vi "JSON_Mass_Find (SubVI).vi"(10 "Array in":string[](array[string]), 11 "Param":string) -> (3 "Array out":string[](array[string]))   [LabVIEW 2018]
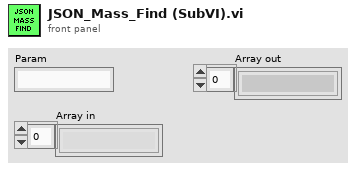
[diagram p1: front panel]
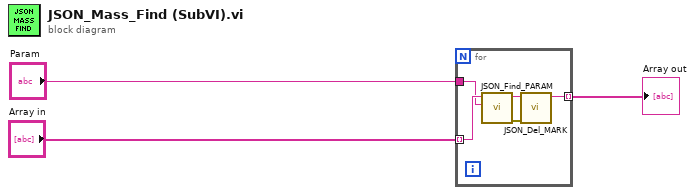
[diagram p0: block diagram]
diagram:
  n1 = for {
    tunnel: "Array in" -> [w8] mode=indexing
    tunnel: [w5] -> w2 mode=indexing
    tunnel: "Param" -> [w4]
    n2 = call "JSON_Find_PARAM.vi"("data"=w4, "name"=w8) -> ("error out"=w6:errorcluster, "String"=w7:string)  [unwired: 8 in]
    n3 = call "JSON_Del_MARK.vi"("error in (no error)"=w6, "String"=w7) -> ("result string"=w5:string)  [unwired: 8 in, 1 out]
  }
  "Array out" <- w2
